vi "Enter_IO.vi"() -> ()   [LabVIEW 2013]
uses:
  <instrlib>/niDMM/nidmm.llb/niDMM Function.ctl
  <instrlib>/niDMM/nidmm.llb/niDMM Resolution in Digits.ctl
  Typedef/event var.ctl
panel:
  in  "Instr. Descriptor (GPIB::30)":string="GPIB::30"
  in  "RUN":bool
  in  "power relay name":refnum<k15>="R_power" caption="resource name"
  in  "Tab Control":T1(tab)
  in  "Volts AC":dbl=120.0
  in  "UUT names 4":string[](array[string])=["UUT1", "UUT2", "UUT3", "UUT4", "UUT5", "UUT6", "UUT7", "UUT8", "UUT9", "UUT10", "UUT11", "UUT12"]
  in  "AC connect relay":bool[](array[boolean])=[FALSE, FALSE, TRUE, TRUE, FALSE, FALSE, FALSE, FALSE, FALSE, FALSE, FALSE, FALSE]
  in  "DC connect relay":bool[](array[boolean])=[FALSE, FALSE, TRUE, TRUE, FALSE, FALSE, FALSE, FALSE, FALSE, FALSE, FALSE, FALSE]
  in  "Volts DC":dbl=24.0
  in  "Cluster":T2
  in  "Timing":T3
  in  "UUT single-ended scan array":T4(array[cluster]) {"Numeric 2" format="%#_3f"}
  in  "UUT names":string[](array[string])=["UUT1", "UUT2", "UUT3", "UUT4", "UUT5", "UUT6", "UUT7", "UUT8", "UUT9", "UUT10", "UUT11", "UUT12"]
  in  "channels":string[](array[string])=["1", "2", "3", "4", "5", "6", "7", "8"]
  in  "UUT names 5":string[](array[string])=["UUT1", "UUT2", "UUT3", "UUT4", "UUT5", "UUT6", "UUT7", "UUT8", "UUT9", "UUT10", "UUT11", "UUT12"]
  in  "Array 3":cluster{"Ring":u16}[][](array[cluster]) {"Ring" items=["None", "MODBUS RTU", "HART (1)", "HART (2)", "Fieldbus", "Profibus DP", "Profibus PA"]}
  out "Oven Air Temperature":dbl(graph)
  in  "stop":bool
  in  "resource name 2":refnum<k15>="DMM" caption="resource name"
  in  "resource name":refnum<k15>="R_signal"
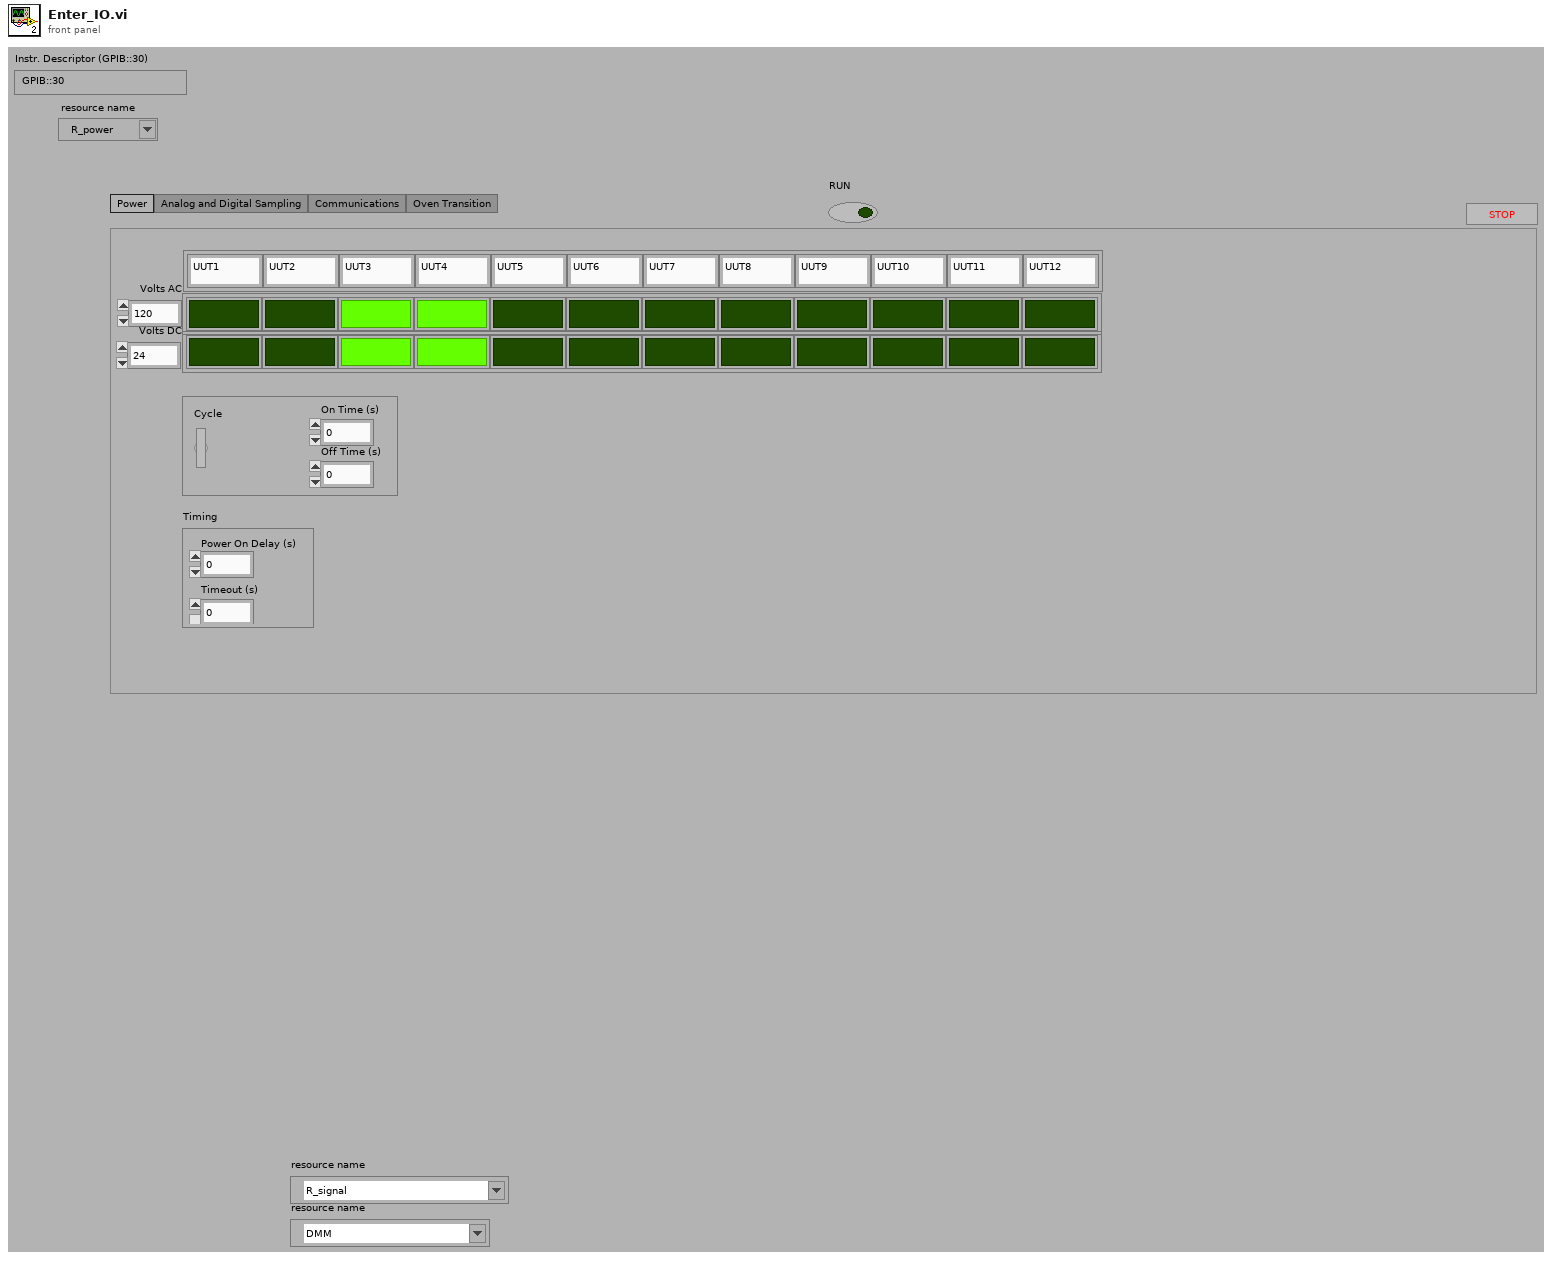
[diagram p1: front panel]
types:
  T1 = enum32{"Power", "Analog and Digital Sampling", "Communications", "Oven Transition"}
  T2 = cluster{"On Time (s)":dbl, "Off Time (s)":dbl, "Cycle":bool}
  T3 = cluster{"Power On Delay (s)":dbl, "Timeout (s)":dbl}
  T4 = cluster{"on?":bool, "Label":string, "measurement type":enum16{"Voltage", "Frequency"}, "Numeric 2":dbl}[][]
  T5 = typedef "event var.ctl" = cluster{"Action":enum16{"Idle", "Update_comm_vars", "DMM_add_data", "Comm_add_data", "Therm_add_data", "Power_add_data", "Update graph", "Write log", "Setup and initialize", "Update Timing vars", "Update status line", "Update config refs"}, "Variant":variant}
  T6 = cluster{"VIRef":refnum<vi>, "PathCurr":path, "Reads":i32, "POWER_QUEUE":refnum<queue>}
  T7 = cluster{"VIRefNm":refnum<vi>, "CurrPath":path, "Results":cluster{"Kc":string, "Cfg":dbl[]}, "DMM_QUEUE":refnum<queue>, "POWER_QUEUE":refnum<queue>}
  T8 = cluster{"VIRef":refnum<vi>, "PathCurr":path, "Reads":i32, "DMM_QUEUE":refnum<queue>}
  T9 = enum16{"Idle", "Update_comm_vars", "DMM_add_data", "Comm_add_data", "Therm_add_data", "Power_add_data", "Update graph", "Write log", "Setup and initialize", "Update Timing vars", "Update status line", "Update config refs"}
  T10 = typedef "niDMM Function.ctl" = enum16{"DC Volts", "AC Volts", "DC Current", "AC Current", "2-wire Resistance", "4-wire Resistance", "Diode", "Frequency", "Period", "AC Volts DC Coupled", "Capacitance", "Inductance", "Temperature"}
  T11 = typedef "niDMM Resolution in Digits.ctl" = dbl
  T12 = cluster{"on?":bool, "Label":string, "measurement type":enum16{"Voltage", "Frequency"}, "Numeric 2":dbl}
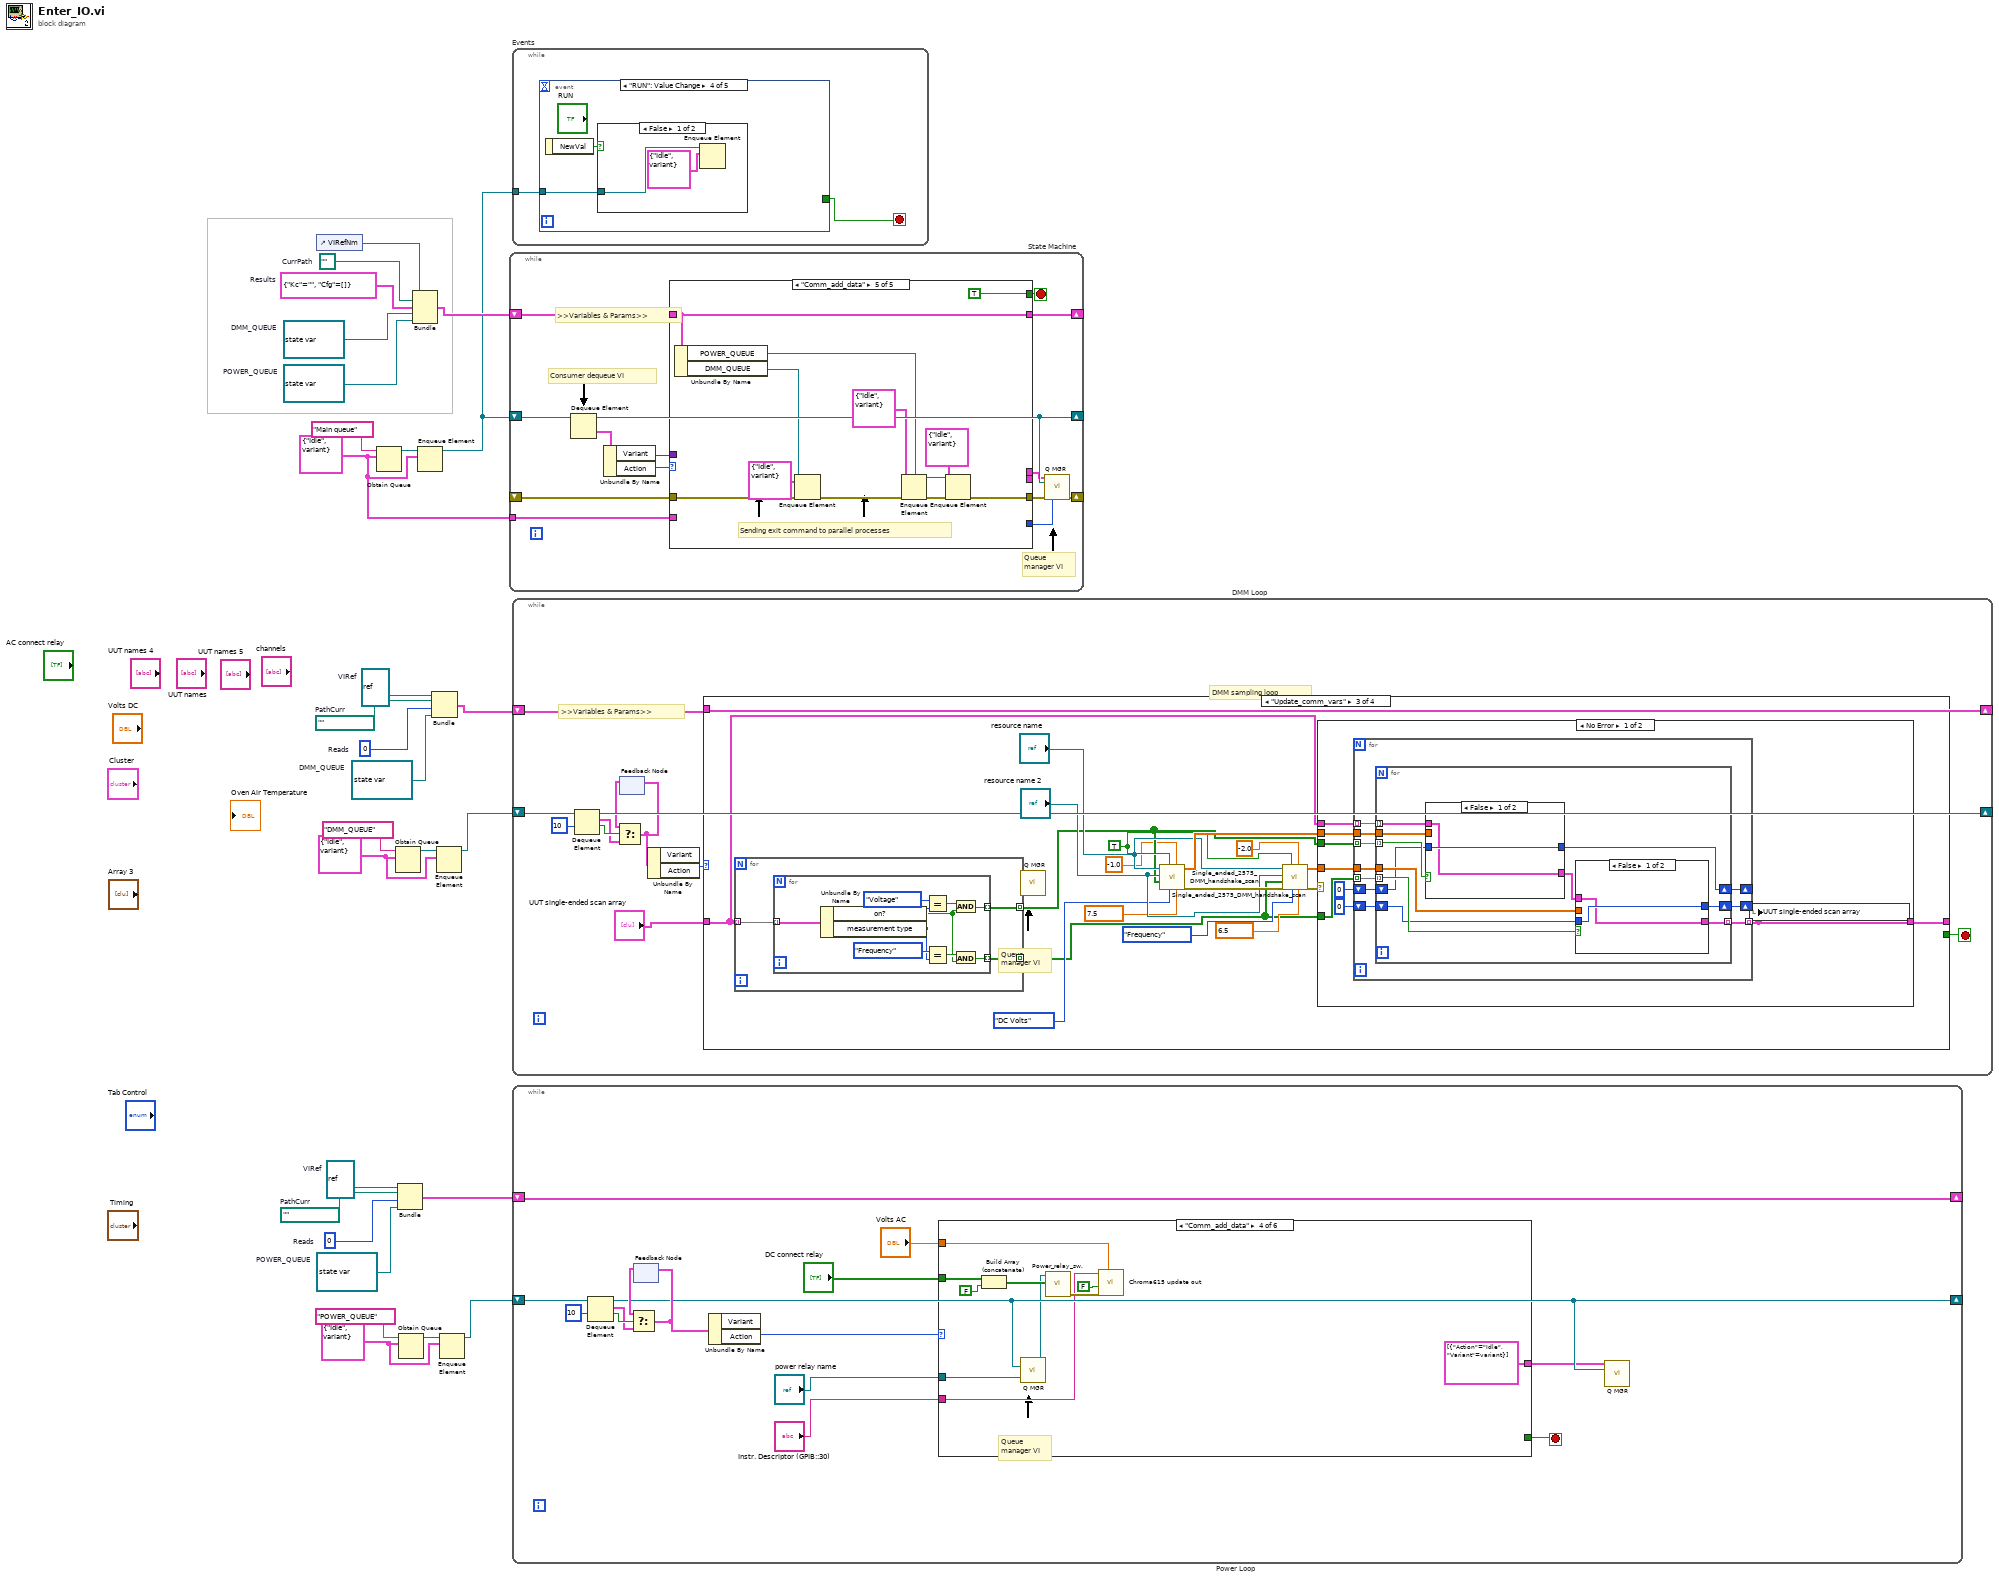
[diagram p0: block diagram]
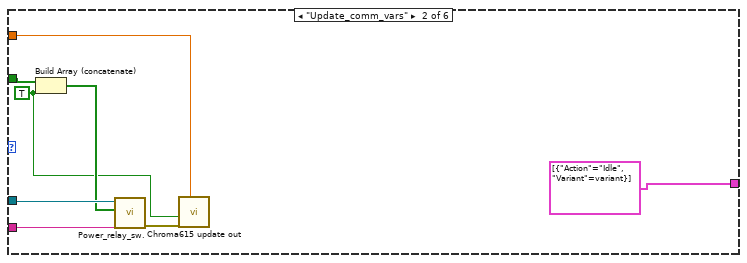
[diagram p3: hidden frame]
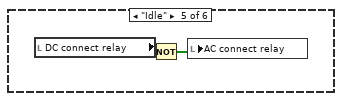
[diagram p5: hidden frame]
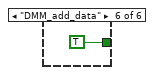
[diagram p6: hidden frame]
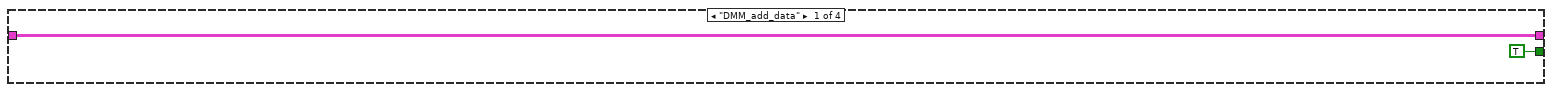
[diagram p7: hidden frame]
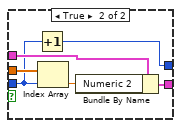
[diagram p9: hidden frame]
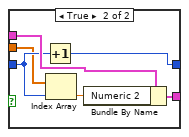
[diagram p10: hidden frame]
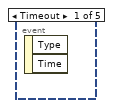
[diagram p13: hidden frame]
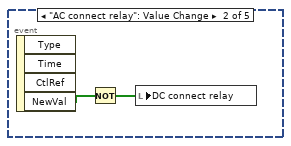
[diagram p14: hidden frame]
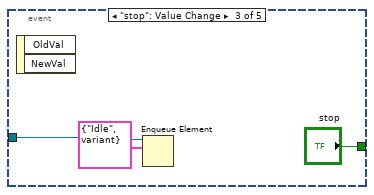
[diagram p15: hidden frame]
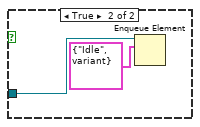
[diagram p16: hidden frame]
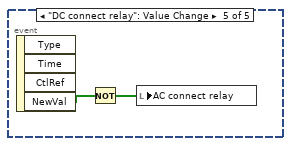
[diagram p17: hidden frame]
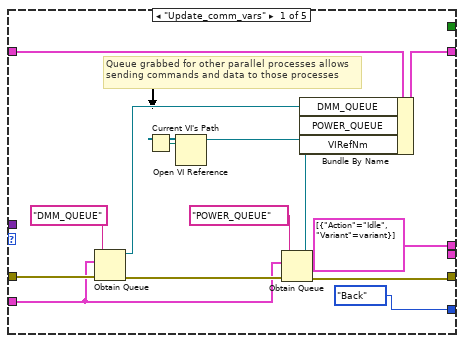
[diagram p18: hidden frame]
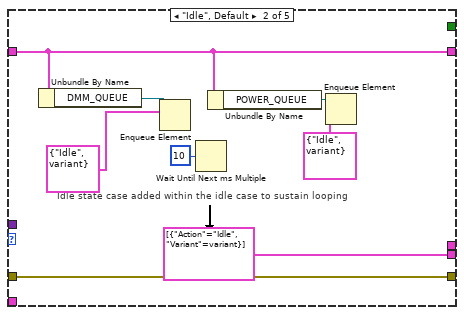
[diagram p19: hidden frame]
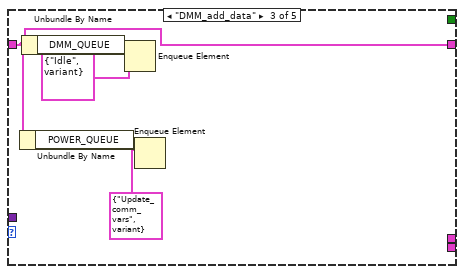
[diagram p20: hidden frame]
diagram:
  w2 = T5 {"Action"=enum."Idle", "Variant"=variant} ("state var")
  w8 = T5 {"Action"=enum."Idle", "Variant"=variant} ("state var")
  w13 = refnum<queue> refnum  # POWER_QUEUE
  w12 = 0  # Reads
  w10 = refnum<vi> refnum  # VIRef
  w11 = path ""  # PathCurr
  w14 = refnum<queue> refnum  # DMM_QUEUE
  w15 = refnum<queue> refnum  # POWER_QUEUE
  w16 = refnum<queue> refnum  # DMM_QUEUE
  w19 = 0  # Reads
  w21 = refnum<vi> refnum  # VIRef
  w20 = path ""  # PathCurr
  w24 = path ""  # CurrPath
  w25 = cluster{"Kc":string, "Cfg":dbl[]} {"Kc"="", "Cfg"=[]}  # Results
  w17 = T5 {"Action"=enum."Idle", "Variant"=variant} ("state var")
  # "DMM sampling loop"
  n1 = control-ref of="VIRefNm"() -> (w26:refnum<vi>)
  n2 = Obtain Queue(name (unnamed)="Main queue", element data type=w17) -> (queue out=w28:refnum<queue>)  [unwired: 3 in, 2 out]
  n3 = Obtain Queue(name (unnamed)="DMM_QUEUE", element data type=w8) -> (queue out=w6:refnum<queue>)  [unwired: 3 in, 2 out]
  n4 = Bundle("VIRef"=w10, "PathCurr"=w11, "Reads"=w12, "POWER_QUEUE"=w13) -> (w9:T6)  [unwired: 1 in]
  n5 = Obtain Queue(name (unnamed)="POWER_QUEUE", element data type=w2) -> (queue out=w4:refnum<queue>)  [unwired: 3 in, 2 out]
  n6 = Bundle("VIRefNm"=w26, "CurrPath"=w24, "Results"=w25, "DMM_QUEUE"=w16, "POWER_QUEUE"=w15) -> (w23:T7)  [unwired: 1 in]
  n7 = Enqueue Element(queue=w28, element=w17) -> (queue out=w22:refnum<queue>)  [unwired: 2 in, 2 out]
  n8 = Bundle("VIRef"=w21, "PathCurr"=w20, "Reads"=w19, "DMM_QUEUE"=w14) -> (w18:T8)  [unwired: 1 in]
  n9 = Enqueue Element(queue=w6, element=w8) -> (queue out=w5:refnum<queue>)  [unwired: 2 in, 2 out]
  n10 = Enqueue Element(queue=w4, element=w2) -> (queue out=w1:refnum<queue>)  [unwired: 2 in, 2 out]
  n11 = while "State Machine" {
    shift-right: [w37] -> _
    shift-left: _ -> [w36]
    shift-right: [w32] -> _
    shift-left: w22 -> [w42]
    shift-right: [w34] -> _
    shift-left: w23 -> [w35]
    tunnel: w17 -> [w31]
    stop <- w29 stop-if-true
    # "Queue manager VI"
    # "Consumer dequeue VI"
    # ">>Variables & Params>>"
    n12 = Dequeue Element(queue=w42) -> (queue out=w32:refnum<queue>, element=w41:T5)  [unwired: 2 in, 2 out]
    n13 = Unbundle By Name(w41) -> ("Variant"=w40:variant, "Action"=w39:T9)
    n14 = case shown="\"Stop\"" w39 {
      tunnel: w36 -> [w49 w64 _ w71 w83]
      tunnel: [w50 w64 _ w70 w81] -> w38
      tunnel: w40 -> [_ _ _ _ _]
      tunnel: [_ T5[] [{"Action"=enum."Idle", "Variant"=variant}] _ _ _] -> _
      tunnel: w35 -> [w56 w60 w67 w72 w80]
      tunnel: [w55 w60 w67 w72 w80] -> w34
      tunnel: [enum16{"Back", "Front", "Replace"}."Back" ("FNs") _ _ _ _] -> w33
      tunnel: w31 -> [w48 _ _ _ _]
      tunnel: [T5[] [{"Action"=enum."Idle", "Variant"=variant}] ("QSTATES") _ _ _ _] -> w30
      tunnel: [_ _ _ _ TRUE] -> w29
      frame "Update_comm_vars" {
        # "Queue grabbed for other parallel processes allows sending commands and data to those processes"
        n15 = Obtain Queue(name (unnamed)="DMM_QUEUE", element data type=w48, error in (no error)=w49) -> (queue out=w47:refnum<queue>, error out=w54:errorcluster)  [unwired: 2 in, 1 out]
        n16 = Current VI's Path() -> (path=w46:path)
        n17 = Open VI Reference(vi path=w46) -> (vi reference=w45:refnum<vi>)  [unwired: 5 in, 1 out]
        n18 = Obtain Queue(name (unnamed)="POWER_QUEUE", element data type=w48, error in (no error)=w54) -> (queue out=w51:refnum<queue>, error out=w50:errorcluster)  [unwired: 2 in, 1 out]
        n19 = Bundle By Name(cluster=w56, "DMM_QUEUE"=w47, "POWER_QUEUE"=w51, "VIRefNm"=w45) -> (w55:T7)
      }
      frame "Idle", Default {
        # "Idle state case added within the idle case to sustain looping"
        n20 = Unbundle By Name(w60) -> ("DMM_QUEUE"=w61:refnum<queue>)
        n21 = Enqueue Element(queue=w61, element=T5 {"Action"=enum."Idle", "Variant"=variant} ("state var")) -> ()  [unwired: 2 in, 3 out]
        n22 = Wait Until Next ms Multiple(millisecond multiple=u32 10) -> ()  [unwired: 1 out]
        n23 = Unbundle By Name(w60) -> ("POWER_QUEUE"=w59:refnum<queue>)
        n24 = Enqueue Element(queue=w59, element=T5 {"Action"=enum."Idle", "Variant"=variant}) -> ()  [unwired: 2 in, 3 out]
      }
      frame "DMM_add_data" {
        n25 = Unbundle By Name(w67) -> ("POWER_QUEUE"=w66:refnum<queue>)
        n26 = Unbundle By Name(w67) -> ("DMM_QUEUE"=w69:refnum<queue>)
        n27 = Enqueue Element(queue=w69, element=T5 {"Action"=enum."Idle", "Variant"=variant}) -> ()  [unwired: 2 in, 3 out]
        n28 = Enqueue Element(queue=w66, element=T5 {"Action"=enum."Update_comm_vars", "Variant"=variant}) -> ()  [unwired: 2 in, 3 out]
      }
      frame "Idle" {
        # "Error Dialog"
        # "Error is cleared after handling"
        n29 = call <vilib>:"Simple Error Handler.vi"("error in (no error)"=w71) -> ()  [unwired: 4 in, 5 out]
        n30 = call "Error Clear.vi"("error in"=w71) -> ("error in (no error)"=w70:errorcluster)  [unwired: 7 in]
      }
      frame "Comm_add_data" {
        # "Sending exit command to parallel processes"
        n31 = Unbundle By Name(w80) -> ("POWER_QUEUE"=w79:refnum<queue>, "DMM_QUEUE"=w78:refnum<queue>)
        n32 = Enqueue Element(queue=w78, element=T5 {"Action"=enum."Idle", "Variant"=variant}, error in (no error)=w83) -> (error out=w82:errorcluster)  [unwired: 1 in, 2 out]
        n33 = Enqueue Element(queue=w79, element=T5 {"Action"=enum."Idle", "Variant"=variant}, error in (no error)=w82) -> (queue out=w74:refnum<queue>, error out=w81:errorcluster)  [unwired: 1 in, 1 out]
        n34 = Enqueue Element(queue=w74, element=T5 {"Action"=enum."Idle", "Variant"=variant}) -> ()  [unwired: 2 in, 3 out]
      }
    }
    n35 = call "Q MGR.vi"("QSTATES"=w30, "Q ref"=w32, "Error IN"=w38, "FNs"=w33) -> ("Error OUT"=w37:errorcluster)  [unwired: 11 in]
  }
  n36 = while "Events" {
    tunnel: w22 -> [w84]
    stop <- w85 stop-if-true
    n37 = event shown="[3] \"RUN\": Value Change" {
      selector: _ -> [_ _ _ _ _]
      dyn-events: _ -> [_ _ _ _ _]
      timeout: _ -> [_ _ _ _ _]
      tunnel: [_ _ "stop" _ _] -> w85
      tunnel: w84 -> [_ _ w88 w91 _]
      event Timeout {
        n38 = event-data() -> ()  [unwired: 1 in, 2 out]
      }
      event "AC connect relay": Value Change {
        n39 = event-data() -> ("NewVal"=w87:bool[])  [unwired: 1 in, 3 out]
        n40 = Not(x=w87) -> (.not. x?=w86:bool[])
        n41 = local write "DC connect relay"(w86) -> ()
      }
      event "stop": Value Change {
        n42 = event-data() -> ()  [unwired: 1 in, 2 out]
        n43 = Enqueue Element(queue=w88, element=T5 {"Action"=enum."Idle", "Variant"=variant} ("event data")) -> ()  [unwired: 2 in, 3 out]
      }
      event "RUN": Value Change {
        n44 = event-data() -> ("NewVal"=w92:bool)  [unwired: 1 in]
        n45 = case shown="False" w92 {
          tunnel: w91 -> [w94 w96]
          frame False {
            n46 = Enqueue Element(queue=w94, element=T5 {"Action"=enum."Idle", "Variant"=variant} ("event data")) -> ()  [unwired: 2 in, 3 out]
          }
          frame True {
            n47 = Enqueue Element(queue=w96, element=T5 {"Action"=enum."Idle", "Variant"=variant} ("event data")) -> ()  [unwired: 2 in, 3 out]
          }
        }
      }
      event "DC connect relay": Value Change {
        n48 = event-data() -> ("NewVal"=w98:bool[])  [unwired: 1 in, 3 out]
        n49 = Not(x=w98) -> (.not. x?=w97:bool[])
        n50 = local write "AC connect relay"(w97) -> ()
      }
    }
  }
  n51 = while "DMM Loop" {
    shift-right: [w104] -> _
    shift-left: w5 -> [w107]
    shift-right: [w106] -> _
    shift-left: w18 -> [w106]
    stop <- w105 stop-if-true
    # "Queue manager VI"
    # ">>Variables & Params>>"
    n52 = Dequeue Element(queue=w107, timeout in ms (-1)=10) -> (queue out=w104:refnum<queue>, element=w101:T5, timed out?=w102:bool)  [unwired: 1 in, 1 out]
    n53 = feedback #1() -> (w100:T5)  [unwired: 1 in]
    n54 = Select(t=w100, s=w102, f=w101) -> (s? t:f=w99:T5)
    n55 = feedback-in #1(w99) -> ()
    n56 = Unbundle By Name(w99) -> ("Action"=w109:T9)  [unwired: 1 out]
    n57 = case shown="\"Running\"" w109 {
      tunnel: [w110 w112 w114 w188] -> _
      tunnel: "UUT single-ended scan array" -> [w110 w112 w113 w188]
      tunnel: [TRUE _ _ _] -> w105
      tunnel: w106 -> [_ _ _ _]
      frame "DMM_add_data" {
      }
      frame "Idle" {
      }
      frame "Update_comm_vars" {
        w118 = T11 7.5 items=["3 1/2"=3.5, "4 1/2"=4.5, "5 1/2"=5.5, "6 1/2"=6.5, "7 1/2"=7.5] ("Resolution in Digits")
        w120 = T11 6.5 items=["3 1/2"=3.5, "4 1/2"=4.5, "5 1/2"=5.5, "6 1/2"=6.5, "7 1/2"=7.5] ("Resolution in Digits")
        w125 = TRUE ("Differential\nMode")
        n58 = for {
          tunnel: w113 -> [w132] mode=indexing
          tunnel: [w131] -> w122 mode=indexing
          tunnel: [w130] -> w117 mode=indexing
          n59 = for {
            tunnel: w132 -> [w141] mode=indexing
            tunnel: [w138] -> w131 mode=indexing
            tunnel: [w133] -> w130 mode=indexing
            n60 = Unbundle By Name(w141) -> ("on?"=w134:bool, "measurement type"=w136:enum16{"Voltage", "Frequency"})
            n61 = Equal?(x=enum16{"Voltage", "Frequency"}."Voltage" ("measurement type"), y=w136) -> (x = y?=w139:bool)
            n62 = Equal?(x=enum16{"Voltage", "Frequency"}."Frequency" ("measurement type"), y=w136) -> (x = y?=w135:bool)
            n63 = And(x=w139, y=w134) -> (x .and. y?=w138:bool)
            n64 = And(x=w135, y=w134) -> (x .and. y?=w133:bool)
          }
        }
        n65 = call "Single_ended_2575_DMM_handshake_scan.vi"("Resolution in Digits"=w118, "range"=-1.0, "measurement type"=niDMM_Function."DC Volts", "Differential\nMode"=w125, "Scan array"=w122, 10:"resource name"="resource name 2", 11:"resource name"="resource name") -> ("error out"=w128:errorcluster, "Measurements 2"=w129:dbl[])  [unwired: 3 in]
        n66 = call "Single_ended_2575_DMM_handshake_scan.vi"("Resolution in Digits"=w120, "range"=-2.0, "measurement type"=niDMM_Function."Frequency", "Differential\nMode"=w125, "error in (no error)"=w128, "Scan array"=w117, 10:"resource name"="resource name 2", 11:"resource name"="resource name") -> ("error out"=w115:errorcluster, "Measurements 2"=w116:dbl[])  [unwired: 2 in]
        n67 = case shown="No Error" w115 {
          tunnel: w113 -> [w149 w187]
          tunnel: w129 -> [w147 _]
          tunnel: w122 -> [w146 _]
          tunnel: w117 -> [w145 _]
          tunnel: w116 -> [w144 _]
          tunnel: [w142 w187] -> w114
          frame No Error {
            n68 = for {
              tunnel: w146 -> [w159] mode=indexing
              tunnel: w149 -> [w158] mode=indexing
              shift-right: [w157] -> _
              shift-left: 0 -> [w156]
              tunnel: w147 -> [w155]
              tunnel: [w154] -> w142 mode=indexing
              tunnel: w145 -> [w153] mode=indexing
              tunnel: w144 -> [w152]
              shift-right: [w150] -> _
              shift-left: 0 -> [w151]
              n69 = for {
                tunnel: w159 -> [w167] mode=indexing
                tunnel: w158 -> [w170] mode=indexing
                shift-right: [w169] -> w157
                shift-left: w156 -> [w162]
                tunnel: w155 -> [w168]
                tunnel: [w163] -> w154 mode=indexing
                tunnel: w153 -> [w166] mode=indexing
                tunnel: w152 -> [w165]
                shift-right: [w160] -> w150
                shift-left: w151 -> [w161]
                n70 = case shown="False" w167 {
                  tunnel: w170 -> [w179 w186]
                  tunnel: [w180 w185] -> w169
                  tunnel: w162 -> [w180 w184]
                  tunnel: w168 -> [_ w183]
                  tunnel: [w179 w181] -> w164
                  frame False {
                  }
                  frame True {
                    n71 = Increment(x=w184) -> (x+1=w185:i32)
                    n72 = Index Array(array=w183, index=w184) -> (element=w182:dbl)
                    n73 = Bundle By Name(cluster=w186, "Numeric 2"=w182) -> (w181:T12)
                  }
                }
                n74 = case shown="False" w166 {
                  tunnel: w164 -> [w171 w178]
                  tunnel: [w172 w177] -> w160
                  tunnel: w161 -> [w172 w173]
                  tunnel: w165 -> [_ w176]
                  tunnel: [w171 w174] -> w163
                  frame False {
                  }
                  frame True {
                    n75 = Increment(x=w173) -> (x+1=w177:i32)
                    n76 = Index Array(array=w176, index=w173) -> (element=w175:dbl)
                    n77 = Bundle By Name(cluster=w178, "Numeric 2"=w175) -> (w174:T12)
                  }
                }
              }
            }
            n78 = local write "UUT single-ended scan array"(w142) -> ()
          }
          frame Error {
          }
        }
      }
      frame "Idle", Default {
      }
    }
    n79 = call "Q MGR.vi"() -> ()  [unwired: 15 in, 1 out]
  }
  n80 = while "Power Loop" {
    shift-right: [w192] -> _
    shift-left: w1 -> [w195]
    shift-right: [w200] -> _
    shift-left: w9 -> [w200]
    stop <- w201 stop-if-true
    # "Queue manager VI"
    n81 = Dequeue Element(queue=w195, timeout in ms (-1)=10) -> (queue out=w192:refnum<queue>, element=w197:T5, timed out?=w198:bool)  [unwired: 1 in, 1 out]
    n82 = feedback #2() -> (w196:T5)  [unwired: 1 in]
    n83 = Select(t=w196, s=w198, f=w197) -> (s? t:f=w194:T5)
    n84 = feedback-in #2(w194) -> ()
    n85 = Unbundle By Name(w194) -> ("Action"=w193:T9)  [unwired: 1 out]
    n86 = case shown="\"Transitioning_from_run_to_idle\"" w193 {
      tunnel: [_ _ _ _ _ TRUE] -> w201
      tunnel: "DC connect relay" -> [_ w210 _ w220 _ _]
      tunnel: "power relay name" -> [_ w211 _ w217 _ _]
      tunnel: [_ T5[] [{"Action"=enum."Idle", "Variant"=variant}] ("QSTATES") _ T5[] [{"Action"=enum."Idle", "Variant"=variant}] ("QSTATES") _ _] -> w191
      tunnel: "Instr. Descriptor (GPIB::30)" -> [_ w206 _ w214 _ _]
      tunnel: "Volts AC" -> [_ w204 _ w212 _ _]
      frame "Idle", Default {
      }
      frame "Update_comm_vars" {
        w205 = TRUE
        n87 = Build Array (concatenate)(w210, w205) -> (w208:bool[])
        n88 = call "Power_relay_sw..vi"("Relay array in"=w208, "resource name"=w211) -> ("error out 2"=w207:errorcluster)  [unwired: 9 in]
        n89 = call "Chroma615 update out.vi"("AC RMS Voltage (100V)"=w204, "error in (no error)"=w207, "Output On/Off (F: OFF)"=w205, "Instr. Descriptor (GPIB::30)"=w206) -> ()  [unwired: 7 in, 1 out]
      }
      frame "Update_comm_vars" {
      }
      frame "Comm_add_data" {
        n90 = Build Array (concatenate)(w220, FALSE) -> (w218:bool[])
        n91 = call "Power_relay_sw..vi"("Relay array in"=w218, "resource name"=w217) -> ("error out 2"=w215:errorcluster)  [unwired: 9 in]
        n92 = call "Chroma615 update out.vi"("AC RMS Voltage (100V)"=w212, "error in (no error)"=w215, "Output On/Off (F: OFF)"=FALSE, "Instr. Descriptor (GPIB::30)"=w214) -> ()  [unwired: 7 in, 1 out]
      }
      frame "Idle" {
        n93 = local read "DC connect relay"() -> (w222:bool[])
        n94 = Not(x=w222) -> (.not. x?=w221:bool[])
        n95 = local write "AC connect relay"(w221) -> ()
      }
      frame "DMM_add_data" {
      }
    }
    n96 = call "Q MGR.vi"("Q ref"=w192) -> ()  [unwired: 14 in, 1 out]
    n97 = call "Q MGR.vi"("QSTATES"=w191, "Q ref"=w192) -> ()  [unwired: 13 in, 1 out]
  }
